vi "Write Outgoing Work Dispatcher.vi"(8 "error in (no error)":errorcluster, 10 "Outgoing Work Dispatcher Queue":refnum<class "Message Enqueuer.lvclass">, 11 "Worker in":refnum<class "Worker.lvclass">) -> (0 "error out":errorcluster, 3 "Worker out":refnum<class "Worker.lvclass">)   [LabVIEW 2023, in "Worker.lvlib" / "Worker.lvclass"]
doc: "Simple accessor method to set the <b>Outgoing Work Dispatcher</b> enqueuer reference of the <b>Worker</b>. \n\nThe enqueuer reference is used by the Worker to queue up a new task to be completed in the next stage of a work pipeline."
uses:
  Worker.lvclass
  <vilib>/ActorFramework/Message Enqueuer/Message Enqueuer.lvclass
  Worker.lvclass/Worker.ctl
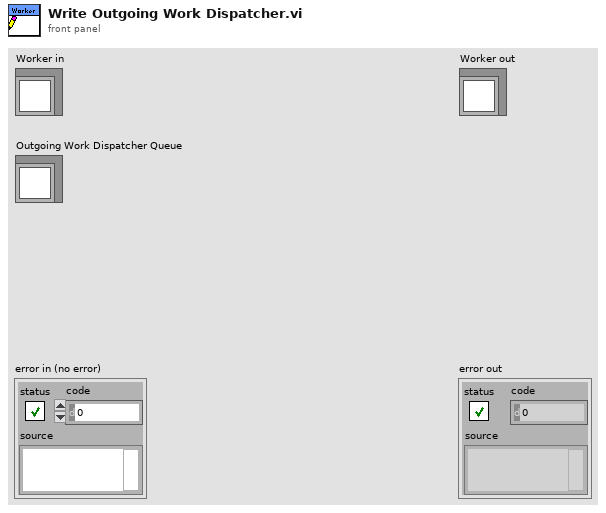
[diagram p1: front panel]
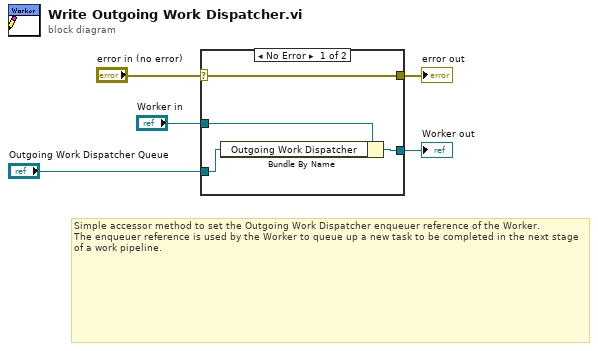
[diagram p0: block diagram]
diagram:
  # "Simple accessor method to set the Outgoing Work Dispatcher enqueuer reference of the Worker.  \nThe enqueuer reference is used by the Worker to queue up a new task to be completed in the next stage of a work pipeline."
  n1 = case shown="No Error" "error in (no error)" {
    selector: "error in (no error)" -> [w9 w10]
    tunnel: [w9 w10] -> w4
    tunnel: [w7 w11] -> w2
    tunnel: "Worker in" -> [w8 w11]
    tunnel: "Outgoing Work Dispatcher Queue" -> [w6 _]
    frame No Error {
      n2 = Bundle By Name(cluster=w8, "Outgoing Work Dispatcher"=w6) -> (w7:refnum<class "Worker.lvclass">)
    }
    frame Error {
    }
  }
  "error out" <- w4
  "Worker out" <- w2
